vi "Read.vi"(8 "error in (no error)":errorcluster caption="错误输入（无错误）", 11 "DMM 输入":refnum<class "DMM.lvclass">) -> (0 "error out":errorcluster caption="错误输出", 2 "Val":dbl, 3 "DMM 输出":refnum<class "DMM.lvclass">)   [LabVIEW 2020, in "DMM.lvlib" / "DMM.lvclass"]
uses:
  DMM.lvclass
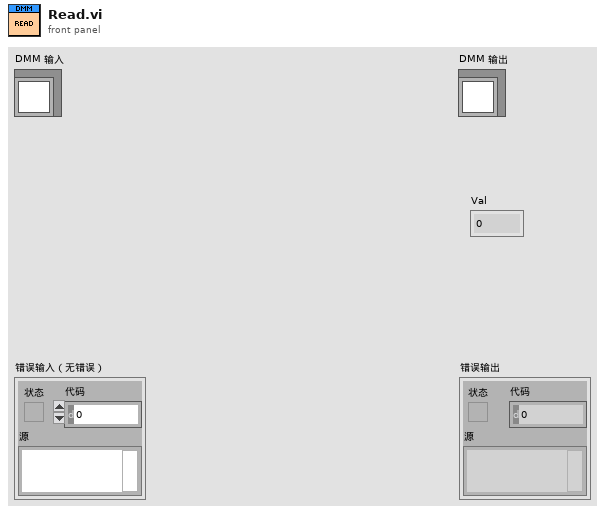
[diagram p1: front panel]
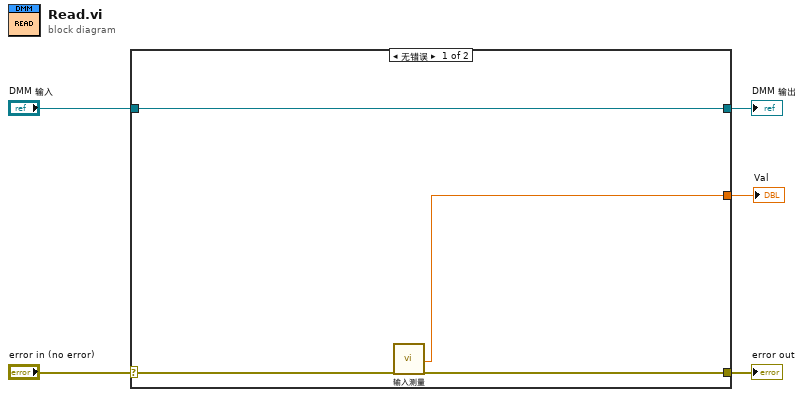
[diagram p0: block diagram]
diagram:
  n1 = case shown="无错误" "error in (no error)" {
    selector: "error in (no error)" -> [w8 w10]
    tunnel: [w7 w10] -> w4
    tunnel: [w9 w11] -> w2
    tunnel: "DMM 输入" -> [w9 w11]
    tunnel: [w6 _] -> w1
    frame No Error {
      n2 = call "输入测量.vi"("error in (no error)"=w8) -> ("数字万用表测量值"=w6:dbl, "error out"=w7:errorcluster)  [unwired: 16 in, 1 out]
    }
    frame Error {
    }
  }
  "error out" <- w4
  "DMM 输出" <- w2
  "Val" <- w1
